vi "PWM_GetValue.vi"(8 "error in":errorcluster, 11 "SonarMB1010DigitalDevRef":T1={"CounterDevRef"={"DevStatus"={"status"=FALSE, "code"=0, "source"=""}, "CntIndex"=enum."Invalid"}, "Scaling factor (s/in)"=0.0}) -> (0 "error out":errorcluster, 2 "Distance":dbl, 3 "SonarMB1010DigitalDevRef":T1={"CounterDevRef"={"DevStatus"={"status"=FALSE, "code"=0, "source"=""}, "CntIndex"=enum."Invalid"}, "Scaling factor (s/in)"=0.0})   [LabVIEW 2017]
doc: "Returns the distance, in inches, between the ultrasonic sensor and the closest object in front of the sensor. The ultrasonic sensor measures this distance by emitting a ping and calculating the time it takes for the echo of the ping to return. If the ultrasonic sensor does not detect the echo of the ping in 50 ms or less, the VI times out and returns a <B>Distance</B> value of 0."
uses:
  <vilib>/Rock Robotics/WPI/Ultrasonic/WPI_SonarMB1010DigitalDeviceRef.ctl
  <vilib>/Rock Robotics/WPI/Counter/WPI_CounterDevRef.ctl
  <vilib>/Rock Robotics/SystemInterfaces/Counter/FPGA_CounterCtrSystemIndex.ctl
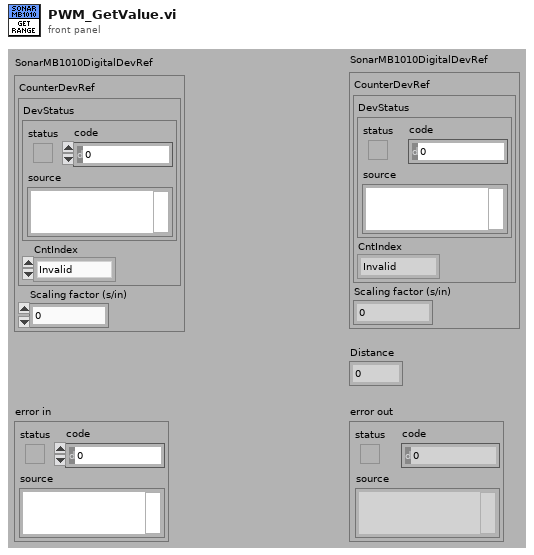
[diagram p1: front panel]
types:
  T1 = typedef "WPI_SonarMB1010DigitalDeviceRef.ctl" = cluster{"CounterDevRef":T2, "Scaling factor (s/in)":dbl}
  T2 = typedef "WPI_CounterDevRef.ctl" = cluster{"DevStatus":errorcluster, "CntIndex":T3}
  T3 = typedef "FPGA_CounterCtrSystemIndex.ctl" = enum8{"Ctr 0", "Ctr 1", "Ctr 2", "Ctr 3", "Ctr 4", "Ctr 5", "Ctr 6", "Ctr 7", "Invalid"}
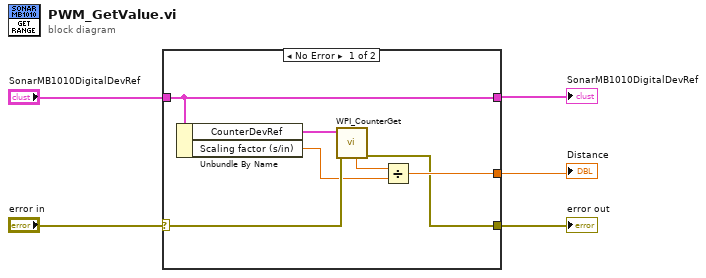
[diagram p0: block diagram]
diagram:
  n1 = case shown="No Error" "error in" {
    selector: "error in" -> [w9 w14]
    tunnel: "SonarMB1010DigitalDevRef" -> [w6 w13]
    tunnel: [w6 w13] -> w3
    tunnel: [w8 w14] -> w4
    tunnel: [w10 _] -> w5
    frame No Error {
      n2 = Unbundle By Name(w6) -> ("CounterDevRef"=w11:T2, "Scaling factor (s/in)"=w7:dbl)
      n3 = call <vilib>:"WPI_CounterGet.vi"("error in (no error)"=w9, "CounterDevRef in"=w11) -> ("error out"=w8:errorcluster, "Period (sec)"=w12:dbl)  [unwired: 4 in, 4 out]
      n4 = Divide(x=w12, y=w7) -> (x/y=w10:dbl)
    }
    frame Error {
    }
  }
  "SonarMB1010DigitalDevRef" <- w3
  "error out" <- w4
  "Distance" <- w5
